vi "cluster_to_byte_data.vi"(1 "element":T1 {"instruction" items=["default"=0, "write"=173, "read"=237, "clear"=205]; "data" format="%x"; "address" format="%x"}) -> (0 "*(type *) &x":string)   [LabVIEW 2018]
uses:
  packet_t.ctl
  packet_type_t.ctl
  spi_instructions.ctl
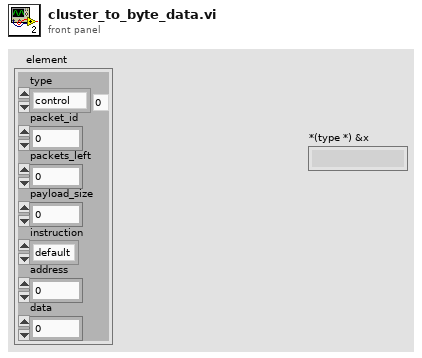
[diagram p1: front panel]
types:
  T1 = typedef "packet_t.ctl" = cluster{"type":T2, "packet_id":u16, "packets_left":u16, "payload_size":u16, "instruction":T3, "address":u8, "data":u8}
  T2 = typedef "packet_type_t.ctl" = enum8{"control", "spi", "audio", "hdmi"}
  T3 = typedef "spi_instructions.ctl" = u8
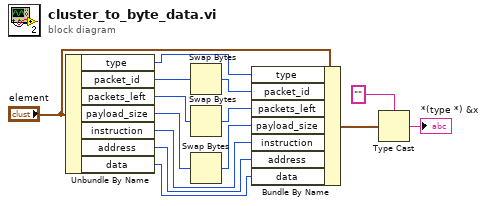
[diagram p0: block diagram]
diagram:
  n1 = Unbundle By Name("element") -> ("type"=w8:T2, "packet_id"=w12:u16, "packets_left"=w11:u16, "payload_size"=w10:u16, "instruction"=w4:T3, "address"=w3:u8, "data"=w2:u8)
  n2 = Swap Bytes(anything=w12) -> (byte swapped=w7:u16)
  n3 = Swap Bytes(anything=w11) -> (byte swapped=w6:u16)
  n4 = Swap Bytes(anything=w10) -> (byte swapped=w5:u16)
  n5 = Bundle By Name(cluster="element", "type"=w8, "packet_id"=w7, "packets_left"=w6, "payload_size"=w5, "instruction"=w4, "address"=w3, "data"=w2) -> (w1:T1)
  n6 = Type Cast(type="" ("data in"), x=w1) -> (*(type *) &x=→"*(type *) &x":string)
